vi "Configure Cycle Count.vi"(8 "error in (no error)":errorcluster, 9 "Cycle Count (1)":i16=1 min=0 max=9999 step=1, 11 "VISA resource name":refnum<visa-resource-name>) -> (0 "error out":errorcluster, 3 "VISA resource name out":refnum<visa-resource-name>)   [LabVIEW 2010, in "Temptronic TP04300.lvlib"]
doc: "This VI writes a cycle count to the TP04300 instrument.\n\n<b>Cycle Count</b> - used to configure the number of cycles.\nConfiguration Parameter Value: this control accepts the cycle count to set the desired number of cycles to run.\n\nDefault Value: 1\nValid Range: 1-9999"
uses:
  Temptronic TP04300.lvlib
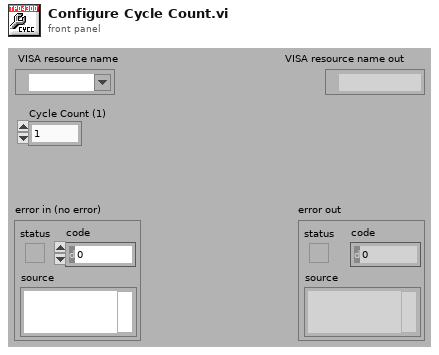
[diagram p1: front panel]
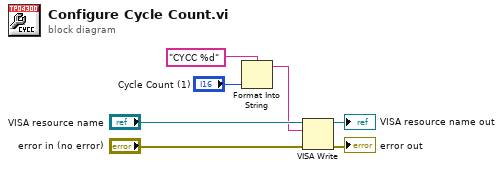
[diagram p0: block diagram]
diagram:
  n1 = Format Into String(format string="CYCC %d", "Cycle Count (1)") -> (resulting string=w3:string)  [unwired: 2 in, 1 out]
  n2 = VISA Write(VISA resource name="VISA resource name", write buffer=w3, error in (no error)="error in (no error)") -> (VISA resource name out=→"VISA resource name out":refnum<visa-resource-name>, error out=→"error out":errorcluster)  [unwired: 1 out]
